vi "Untitled 1.vi"() -> ()   [LabVIEW 2015]
panel:
  out "# Sel Wfms":i32
  out "# Avail Wfms":i32
  in  "Remove":bool
  out "error out":errorcluster
  in  "stop":bool
  in  "Add":bool
  in  "Waveforms to Process":i32[](listbox)
  in  "Available Waveforms":i32[](listbox)
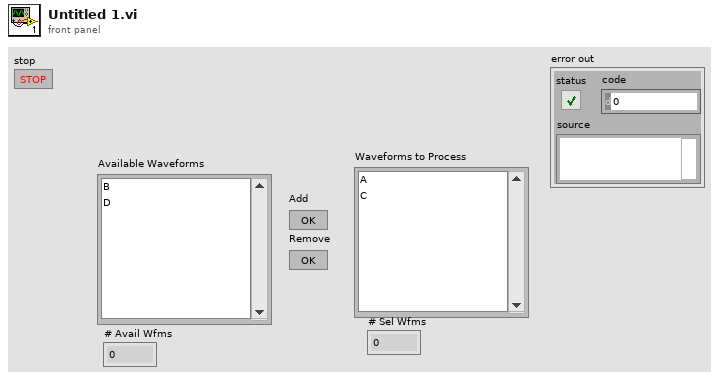
[diagram p1: front panel]
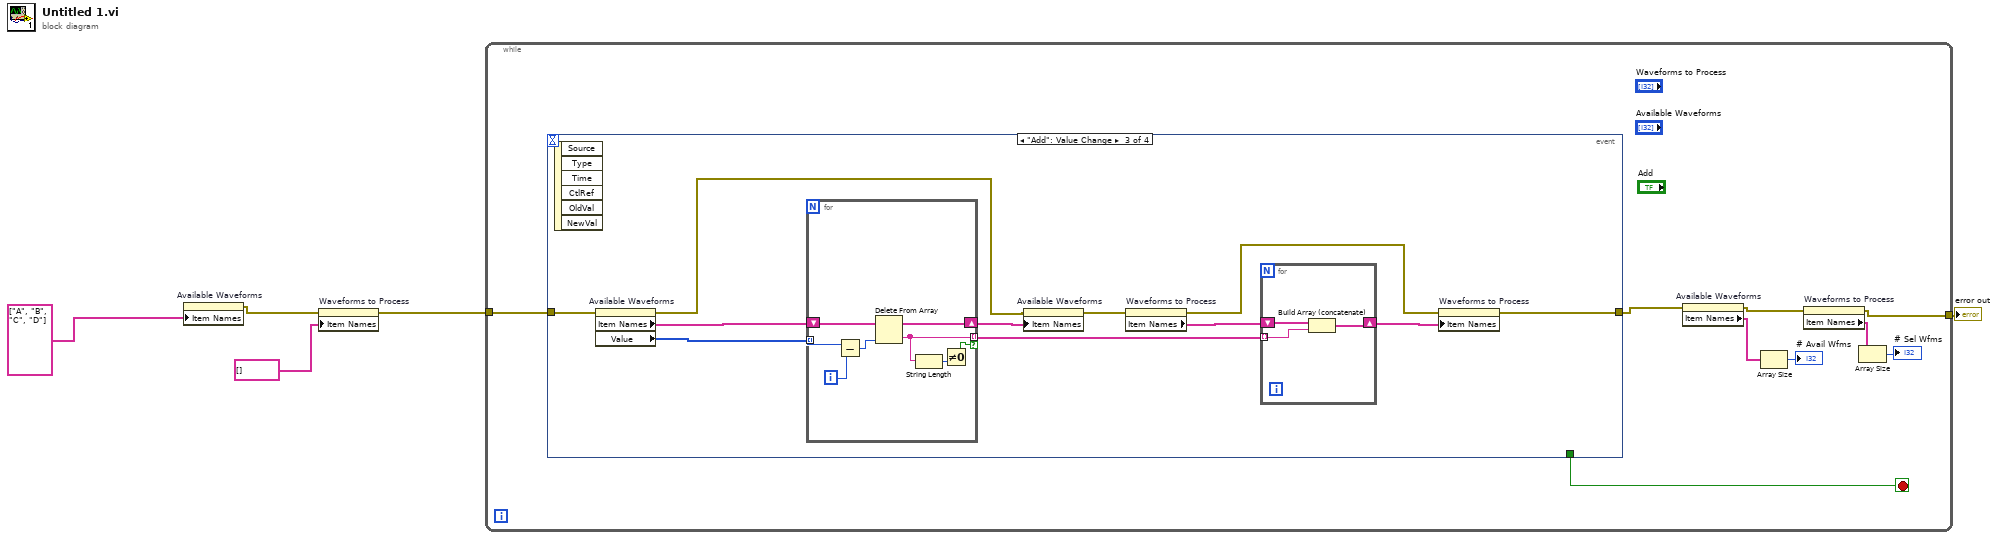
[diagram p0: block diagram]
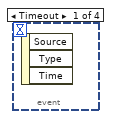
[diagram p2: hidden frame]
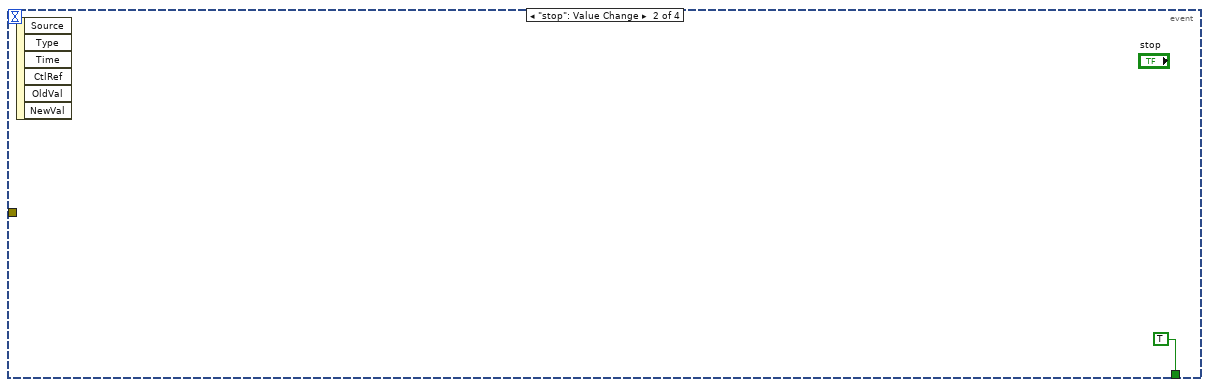
[diagram p3: hidden frame]
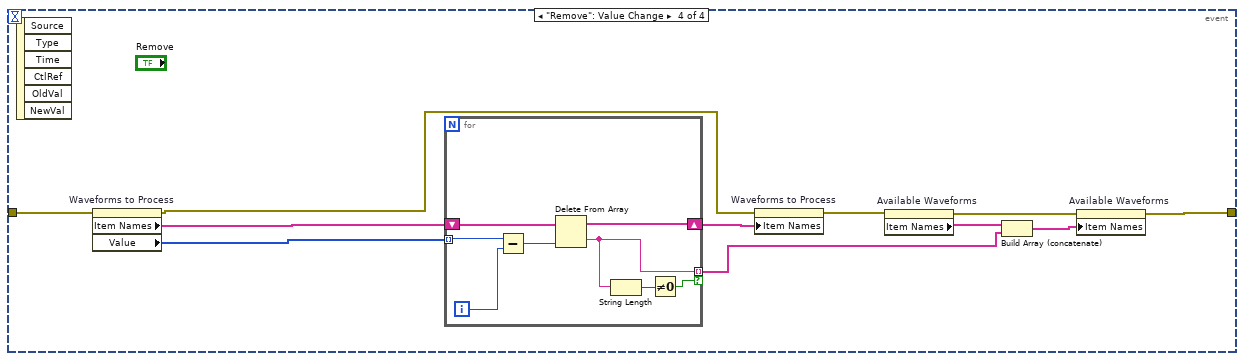
[diagram p4: hidden frame]
diagram:
  n1 = property on="Available Waveforms" class="LstBox (strict)"("Item Names"=string[] ["A", "B", "C", "D"]) -> (error out=w3:errorcluster)  [unwired: 2 in, 1 out]
  n2 = property on="Waveforms to Process" class="LstBox (strict)"(error in=w3, "Item Names"=string[] []) -> (error out=w2:errorcluster)  [unwired: 1 in, 1 out]
  n3 = while {
    tunnel: w2 -> [w13]
    tunnel: [w10] -> w1
    stop <- w14 stop-if-true
    n4 = event shown="[2] \"Add\": Value Change" {
      selector: _ -> [_ _ _ _]
      dyn-events: _ -> [_ _ _ _]
      timeout: _ -> [_ _ _ _]
      tunnel: [_ TRUE _ _] -> w14
      tunnel: w13 -> [_ _ w26 w48]
      tunnel: [_ _ w24 w46] -> w12
      event Timeout {
        n5 = event-data() -> ()  [unwired: 1 in, 3 out]
      }
      event "stop": Value Change {
        n6 = event-data() -> ()  [unwired: 1 in, 6 out]
      }
      event "Add": Value Change {
        n7 = event-data() -> ()  [unwired: 1 in, 6 out]
        n8 = property on="Available Waveforms" class="LstBox (strict)"(error in=w26) -> (error out=w25:errorcluster, "Item Names"=w23:string[], "Value"=w22:i32[])  [unwired: 1 in, 1 out]
        n9 = for {
          tunnel: w22 -> [w36] mode=indexing
          tunnel: [w32] -> w19 mode=indexing if=w30
          shift-right: [w33] -> w16
          shift-left: w23 -> [w37]
          i -> [w35]
          n10 = Subtract(x=w36, y=w35) -> (x-y=w34:i32)
          n11 = Delete From Array(array=w37, index=w34) -> (deleted portion=w32:string, array with subset deleted=w33:string[])  [unwired: 1 in]
          n12 = String Length(string=w32) -> (length=w31:i32)
          n13 = Not Equal To 0?(x=w31) -> (x != 0?=w30:bool)
        }
        n14 = property on="Available Waveforms" class="LstBox (strict)"(error in=w25, "Item Names"=w16) -> (error out=w21:errorcluster)  [unwired: 1 in, 1 out]
        n15 = property on="Waveforms to Process" class="LstBox (strict)"(error in=w21) -> (error out=w18:errorcluster, "Item Names"=w20:string[])  [unwired: 1 in, 1 out]
        n16 = for {
          tunnel: w19 -> [w28] mode=indexing
          shift-right: [w27] -> w17
          shift-left: w20 -> [w29]
          n17 = Build Array (concatenate)(w29, w28) -> (w27:string[])
        }
        n18 = property on="Waveforms to Process" class="LstBox (strict)"(error in=w18, "Item Names"=w17) -> (error out=w24:errorcluster)  [unwired: 1 in, 1 out]
      }
      event "Remove": Value Change {
        n19 = event-data() -> ()  [unwired: 1 in, 6 out]
        n20 = property on="Waveforms to Process" class="LstBox (strict)"(error in=w48) -> (error out=w47:errorcluster, "Item Names"=w45:string[], "Value"=w44:i32[])  [unwired: 1 in, 1 out]
        n21 = for {
          tunnel: w44 -> [w54] mode=indexing
          shift-right: [w56] -> w43
          shift-left: w45 -> [w55]
          tunnel: [w51] -> w40 mode=indexing if=w49
          i -> [w53]
          n22 = Subtract(x=w54, y=w53) -> (x-y=w52:i32)
          n23 = Delete From Array(array=w55, index=w52) -> (deleted portion=w51:string, array with subset deleted=w56:string[])  [unwired: 1 in]
          n24 = String Length(string=w51) -> (length=w50:i32)
          n25 = Not Equal To 0?(x=w50) -> (x != 0?=w49:bool)
        }
        n26 = property on="Waveforms to Process" class="LstBox (strict)"(error in=w47, "Item Names"=w43) -> (error out=w42:errorcluster)  [unwired: 1 in, 1 out]
        n27 = property on="Available Waveforms" class="LstBox (strict)"(error in=w42) -> (error out=w38:errorcluster, "Item Names"=w41:string[])  [unwired: 1 in, 1 out]
        n28 = Build Array (concatenate)(w41, w40) -> (w39:string[])
        n29 = property on="Available Waveforms" class="LstBox (strict)"(error in=w38, "Item Names"=w39) -> (error out=w46:errorcluster)  [unwired: 1 in, 1 out]
      }
    }
    n30 = property on="Available Waveforms" class="LstBox (strict)"(error in=w12) -> (error out=w11:errorcluster, "Item Names"=w9:string[])  [unwired: 1 in, 1 out]
    n31 = Array Size(array=w9) -> (size(s)=→"# Avail Wfms":i32)
    n32 = property on="Waveforms to Process" class="LstBox (strict)"(error in=w11) -> (error out=w10:errorcluster, "Item Names"=w8:string[])  [unwired: 1 in, 1 out]
    n33 = Array Size(array=w8) -> (size(s)=→"# Sel Wfms":i32)
  }
  "error out" <- w1
